vi "EditOptions.vi"(8 "error in":errorcluster, 11 "Simple Sequencer TBM editor node in":refnum<class "Simple Sequencer TBM editor node.lvclass">) -> (0 "error out":errorcluster, 1 "edit options":T1, 2 "subnodes class":T2, 3 "Simple Sequencer TBM editor node out":refnum<class "Simple Sequencer TBM editor node.lvclass">)   [LabVIEW 2015, in "Simple Sequencer TBM editor node.lvclass"]
doc: "This VI Contains the options for the Menu that will be displayed when doing right click on an item\nThe subnodes class configures which nodes can be added to this nodes\nAnd the edit options determine which options are available for the node.\n\nThis configuration is stored in this VI in case some dynamic configuration is required for the menu options or subnodes.\n\nAll VIs must overide this method"
uses:
  Simple Sequencer TBM editor node.lvclass
  <vilib>/NI/Configuration Framework/Node/SubNodeCluster.ctl
  <vilib>/NI/Configuration Framework/Node/NodeMenuOptions.ctl
  <vilib>/NI/Configuration Framework/Node/NISE_CEF_Node.lvclass
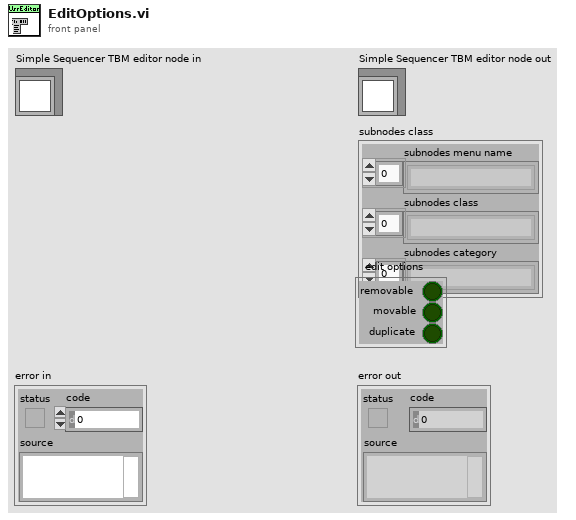
[diagram p1: front panel]
types:
  T1 = typedef "NISE_CEF_Node.lvclass/NodeMenuOptions.ctl" = cluster{"removable":bool, "movable":bool, "duplicate":bool}
  T2 = typedef "NISE_CEF_Node.lvclass/SubNodeCluster.ctl" = cluster{"subnodes menu name":string[], "subnodes class":string[], "subnodes category":string[]}
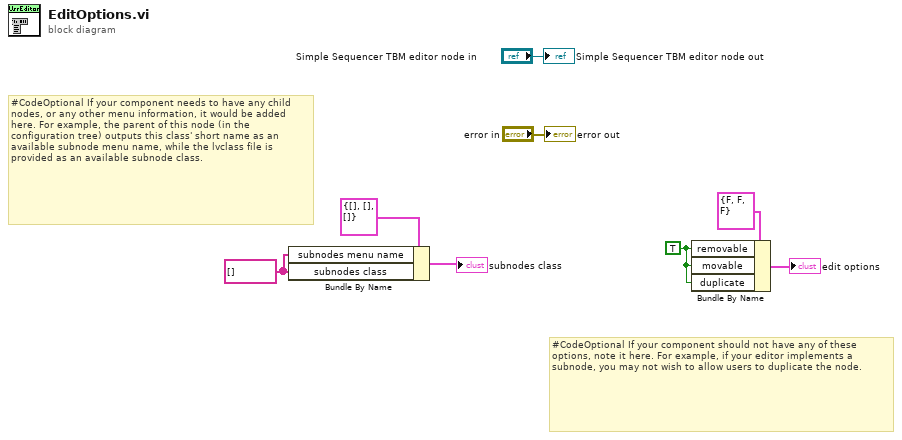
[diagram p0: block diagram]
diagram:
  w3 = TRUE ("removable")
  w4 = string[] [] ("subnodes menu name")
  # "#CodeOptional If your component should not have any of these options, note it here. For example, if your editor implements a subnode, you may not wish to allow users to duplicate the node."
  # "#CodeOptional If your component needs to have any child nodes, or any other menu information, it would be added here. For example, the parent of this node (in the configuration tree) outputs this class' short name as an available subnode menu name, while the lvclass file is provided as an available subnode class."
  n1 = Bundle By Name(cluster=T2 {"subnodes menu name"=[], "subnodes class"=[], "subnodes category"=[]} ("subnodes class"), "subnodes menu name"=w4, "subnodes class"=w4) -> (→"subnodes class":T2)
  n2 = Bundle By Name(cluster=T1 {"removable"=FALSE, "movable"=FALSE, "duplicate"=FALSE} ("edit options"), "removable"=w3, "movable"=w3, "duplicate"=w3) -> (→"edit options":T1)
  "error out" <- "error in"
  "Simple Sequencer TBM editor node out" <- "Simple Sequencer TBM editor node in"
